vi "Read Nulls as Defaults.vi"(8 "error in (no error)":errorcluster, 11 "JSON Deserializer in":refnum<class "JSON Deserializer.lvclass">) -> (0 "error out":errorcluster, 2 "Nulls as Defaults":bool=TRUE, 3 "JSON Deserializer out":refnum<class "JSON Deserializer.lvclass">)   [LabVIEW 2019, in "JKI JSON Serialization.lvlib" / "JSON Deserializer.lvclass"]
doc: "JKI JSON 1.1.10.37\nTomi Maila - JKI\nCopyright (c) 2017, JKI"
uses:
  JSON Deserializer.lvclass
  JSON Deserializer.lvclass/JSON Deserializer.ctl
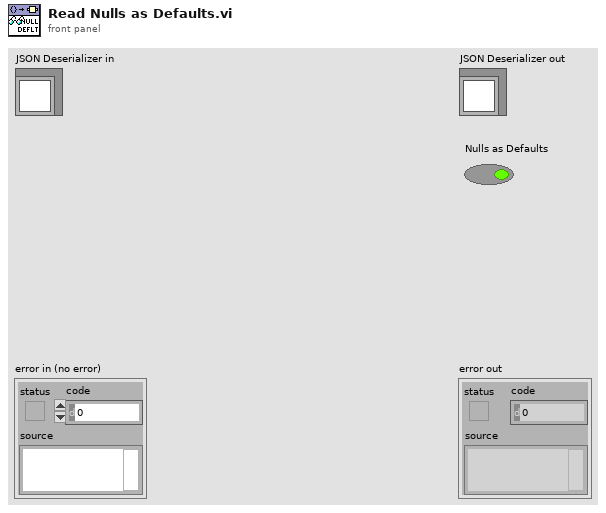
[diagram p1: front panel]
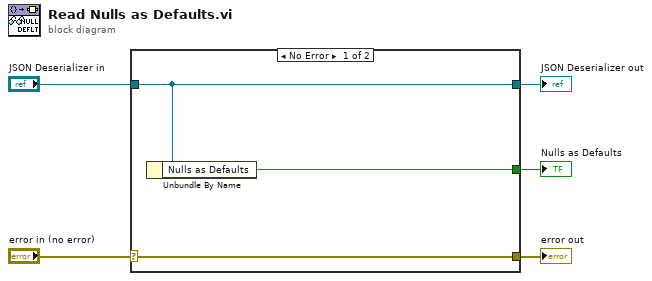
[diagram p0: block diagram]
diagram:
  n1 = case shown="No Error" "error in (no error)" {
    selector: "error in (no error)" -> [w8 w9]
    tunnel: [w8 w9] -> w4
    tunnel: [w7 w10] -> w2
    tunnel: "JSON Deserializer in" -> [w7 w10]
    tunnel: [w6 _] -> w1
    frame No Error {
      n2 = Unbundle By Name(w7) -> ("Nulls as Defaults"=w6:bool)
    }
    frame Error {
    }
  }
  "error out" <- w4
  "JSON Deserializer out" <- w2
  "Nulls as Defaults" <- w1
